vi "Send Command.vi"(8 "error in (no error)":errorcluster, 10 "Consumer Queues in":T1, 11 "UI Process Command in":refnum<class "Generic UI Process Command.lvclass">) -> (0 "error out":errorcluster, 2 "Consumer Queues out":T1)   [LabVIEW 2019, in "User Interface Process.lvlib" / "Generic UI Process Command.lvclass"]
uses:
  Generic UI Process Command.lvclass
  TS Framework/Consumer Queues.ctl
  DAC Process/Generic DAC Command/Generic DAC Process Command.lvclass
  Trig Process/Generic Trig Command/Generic Trig Process Command.lvclass
  TS Framework/TS Framework.lvlib
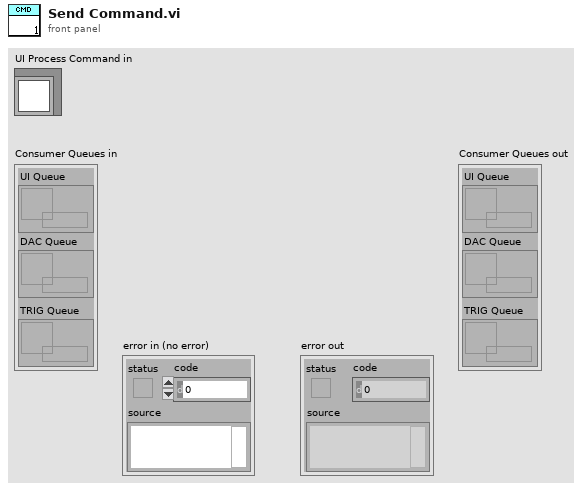
[diagram p1: front panel]
types:
  T1 = typedef "TS Framework.lvlib/Consumer Queues.ctl" = cluster{"UI Queue":refnum<queue>, "DAC Queue":refnum<queue>, "TRIG Queue":refnum<queue>}
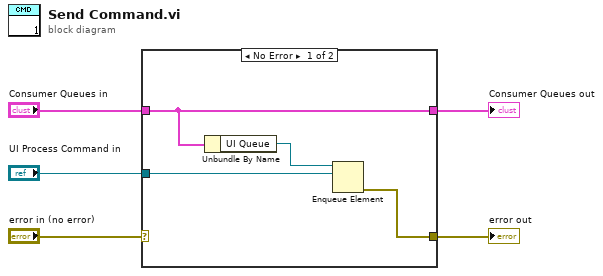
[diagram p0: block diagram]
diagram:
  n1 = case shown="No Error" "error in (no error)" {
    selector: "error in (no error)" -> [_ w11]
    tunnel: "Consumer Queues in" -> [w6 w10]
    tunnel: "UI Process Command in" -> [w8 _]
    tunnel: [w7 w11] -> w3
    tunnel: [w6 w10] -> w1
    frame No Error {
      n2 = Unbundle By Name(w6) -> ("UI Queue"=w9:refnum<queue>)
      n3 = Enqueue Element(queue=w9, element=w8) -> (error out=w7:errorcluster)  [unwired: 2 in, 2 out]
    }
    frame Error {
    }
  }
  "error out" <- w3
  "Consumer Queues out" <- w1
